vi "Tag to Tree ID and Attribute Name.vi"(11 "Tag":string) -> (1 "Attribute Name":string, 2 "Tree ID":string, 3 "Tree":bool)   [LabVIEW 2020, in "NI_VIAnCFGDataStructure.lvlib" / "Tree.lvclass"]
doc: "Convert the Tag returned from Tree Control element to a Tree ID and Attribute Name. The Tree Element boolean output returns True if the Tag looks like a Tree ID and a False if it looks like a Tree ID and Attribute Name."
uses:
  <vilib>/addons/analyzer/VIAnCFGDataStructure/Tree Manager/Tree.lvclass
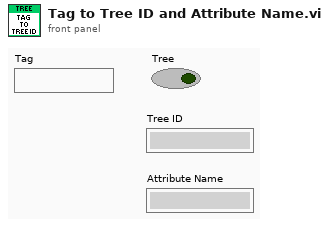
[diagram p1: front panel]
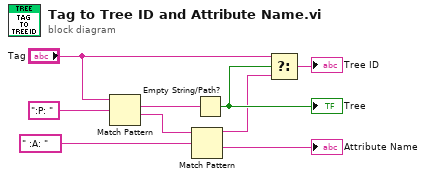
[diagram p0: block diagram]
diagram:
  n1 = Match Pattern(string="Tag", regular expression=":P: " ("string")) -> (match substring=w6:string, after substring=w7:string)  [unwired: 1 in, 2 out]
  n2 = Match Pattern(string=w7, regular expression=" :A: " ("string")) -> (before substring=w1:string, after substring=→"Attribute Name":string)  [unwired: 1 in, 2 out]
  n3 = Empty String/Path?(string/path=w6) -> (empty?=w4:bool)
  "Tree" <- w4
  n4 = Select(t="Tag", s=w4, f=w1) -> (s? t:f=→"Tree ID":string)
